vi "xml generate for SFP+_VNA_Full.vi"(0 "xmlPath":path=path "D:/wmgxml.xml", 5 "txtPath":path, 7 "singleItemInfo":T3[](array[typedef]), 9 "xml_detail":T2, 11 "TDD":T1) -> ()   [LabVIEW 2011]
uses:
  dataType/sSpec.ctl
  dataType/xml_detail.ctl
  dataType/TDD.ctl
  <vilib>/Utility/file.llb/Read From Spreadsheet File (DBL).vi
panel:
  out "FilePath":string
  out "FileVer":string
  out "Limit_NEXT":dbl[](array[numeric])
  out "Limit_SCC11":dbl[](array[numeric])
  out "Limit_SCD21-SDD21":dbl[](array[numeric])
  out "Limit_ILD":dbl[](array[numeric])
  out "Limit_SDD11":dbl[](array[numeric])
  out "limit_SDD21":dbl[](array[numeric])
  out "show_impspec":string[](array[string])
  out "terminal points 2":dbl[](array[numeric])
  in  "width2":dbl
  in  "width1":dbl
  out "TestResult":string
  out "cable points":dbl[](array[numeric])
  out "terminal points":dbl[](array[numeric])
  out "TDD":string
  out "NEXT":string
  out "SCC11":string
  out "SCD21-SDD21":string
  out "ILD":string
  out "SDD11":string
  out "SDD21":string
  out "midVar_time":string[](array[string])
  out "input_array_time":string[](array[string])
  out "input_str_CustomerPN":string
  in  "midVar_state":string
  in  "input_str_product":string
  out "input_str_label":string
  out "midVar_Content":string
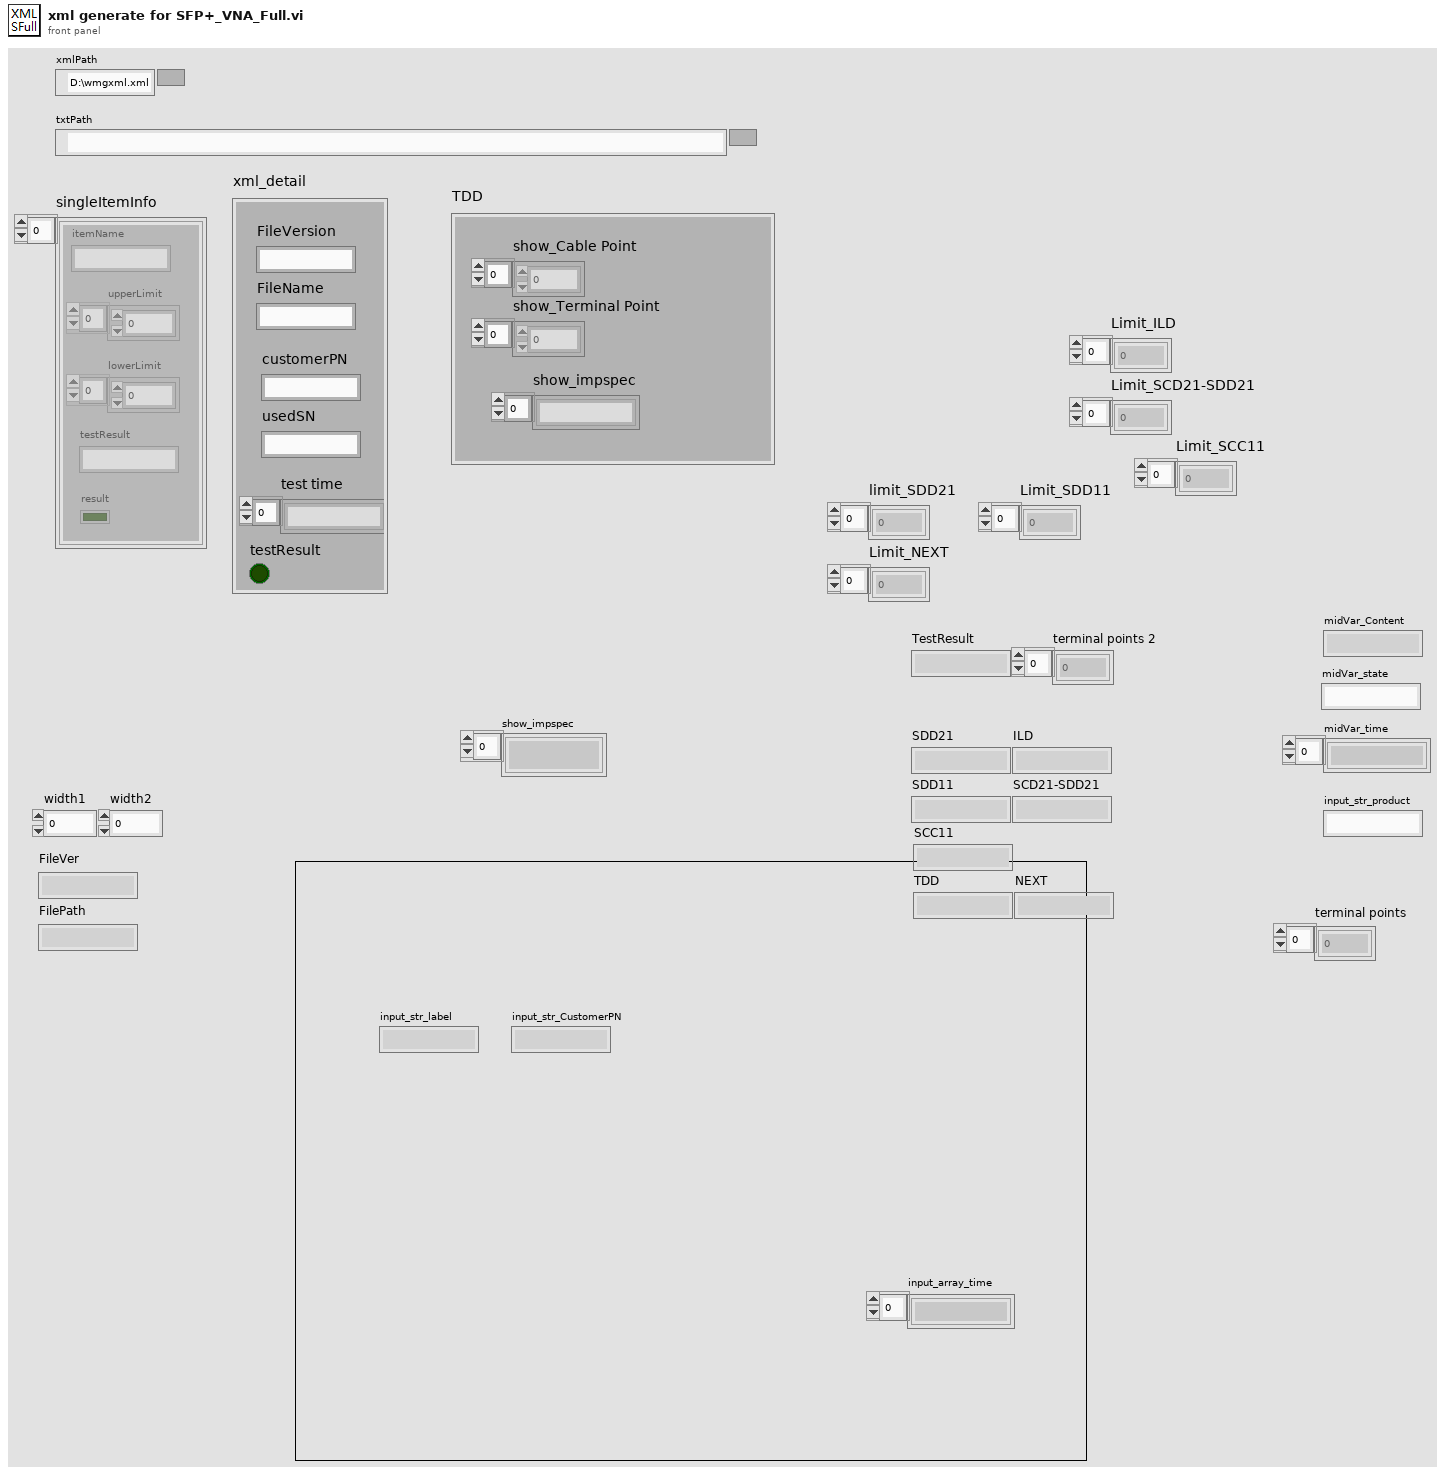
[diagram p1: front panel]
types:
  T1 = typedef "TDD.ctl" = cluster{"show_Cable Point":dbl[], "show_Terminal Point":dbl[], "show_impspec":string[]}
  T2 = typedef "xml_detail.ctl" = cluster{"FileVersion":string, "FileName":string, "customerPN":string, "usedSN":string, "test time":string[], "testResult":bool}
  T3 = typedef "sSpec.ctl" = cluster{"itemName":string, "upperLimit":dbl[], "lowerLimit":dbl[], "testResult":string, "result":bool}
  T4 = enum16{"open", "replace", "create", "open or create", "replace or create", "replace or create with confirmation"}
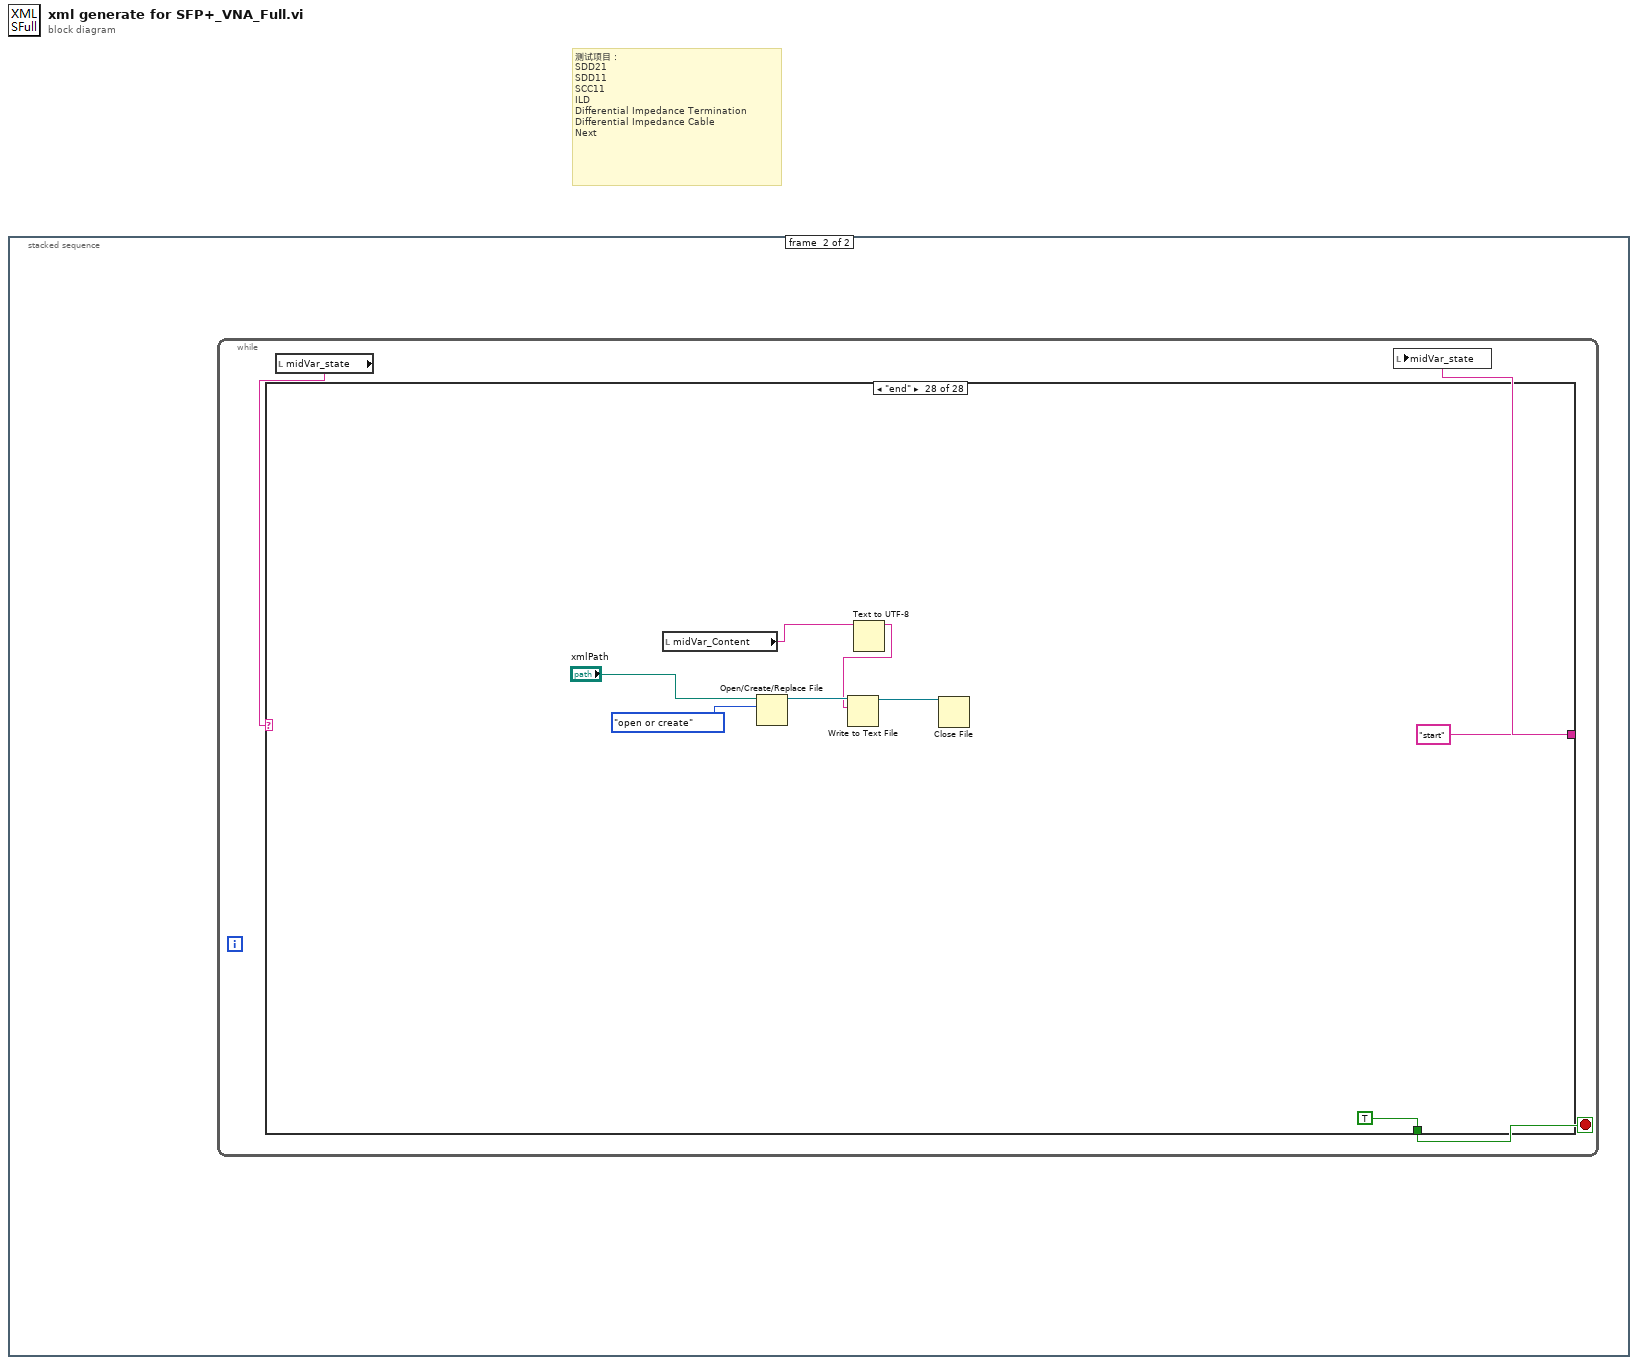
[diagram p0: block diagram]
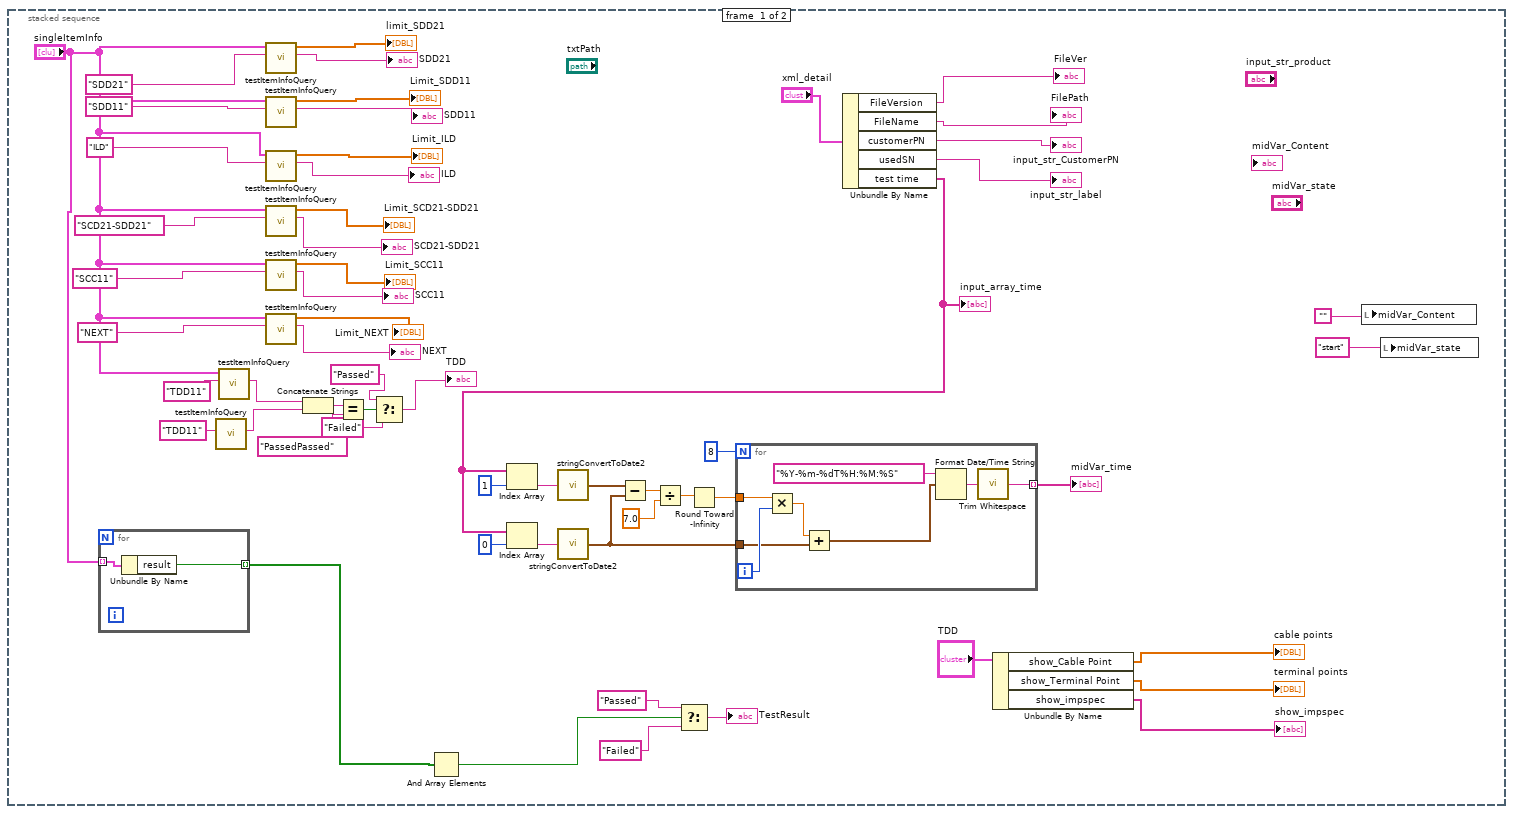
[diagram p2: hidden frame]
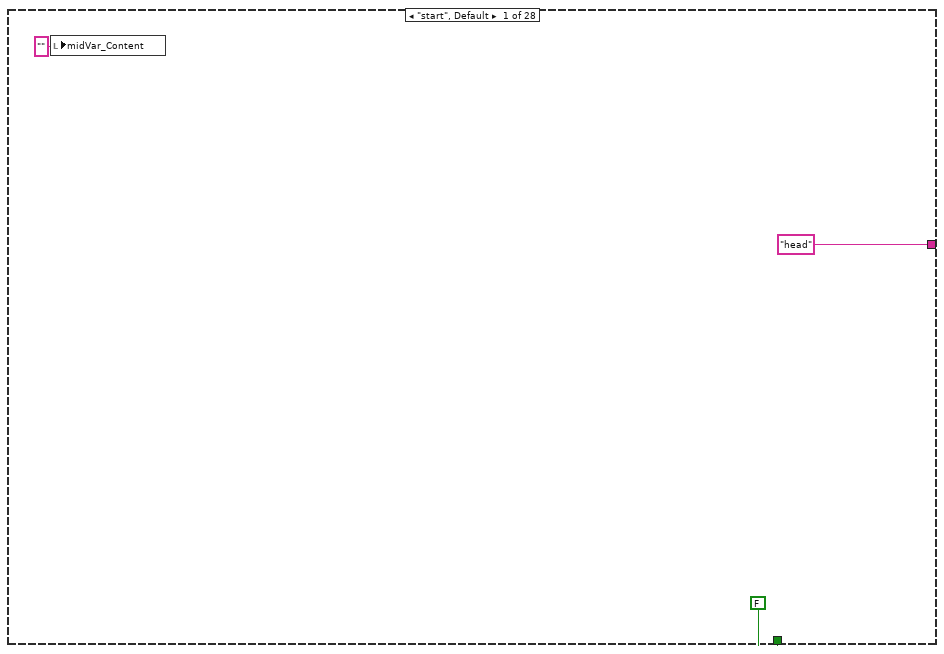
[diagram p3: hidden frame]
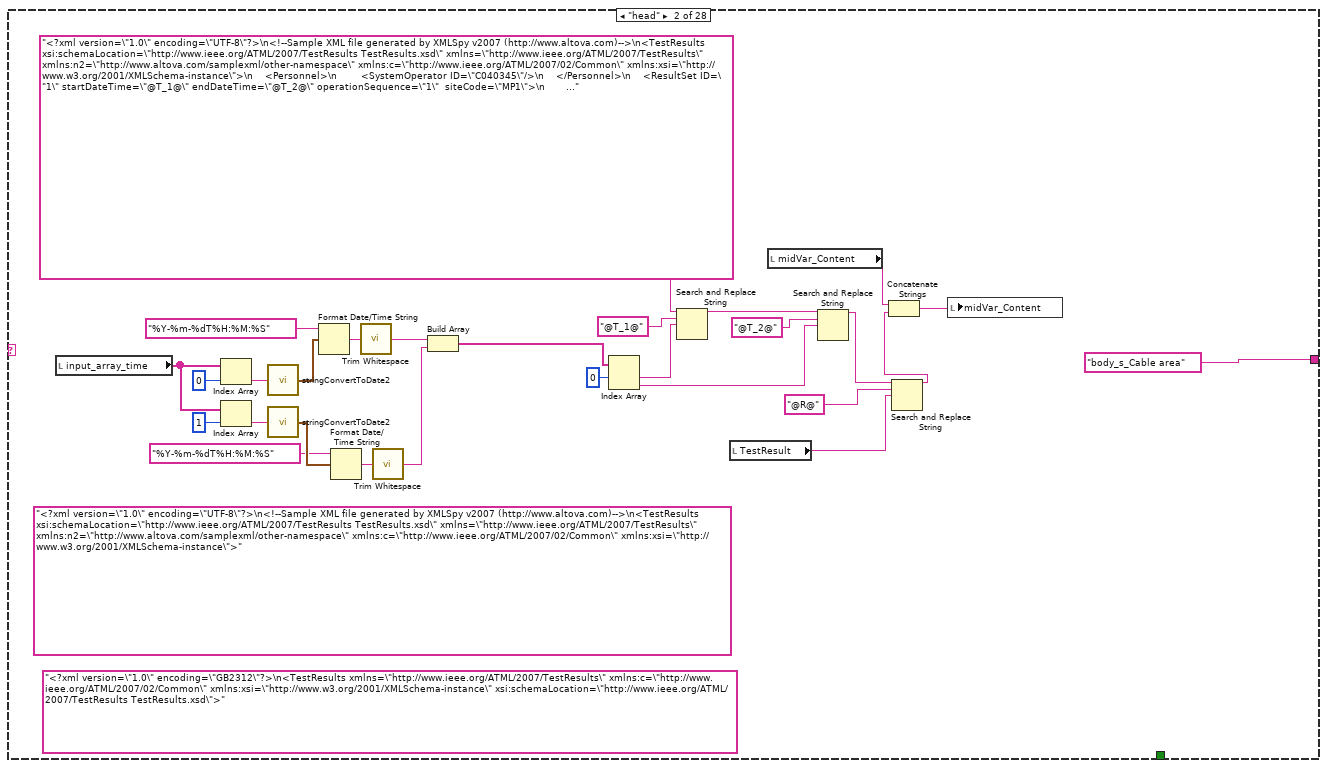
[diagram p4: hidden frame]
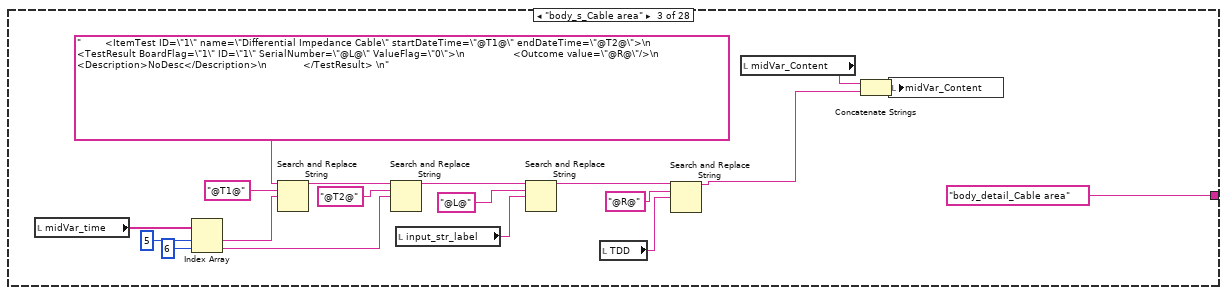
[diagram p5: hidden frame]
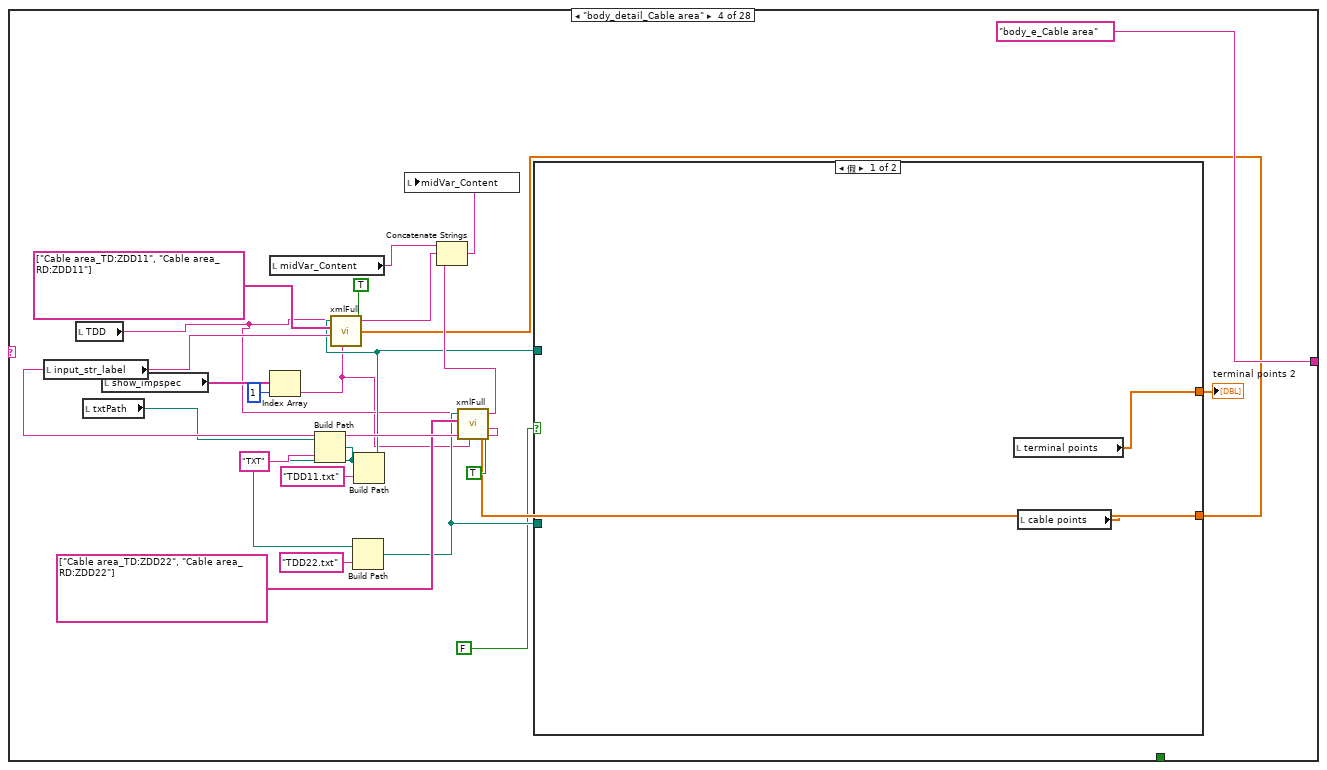
[diagram p6: hidden frame]
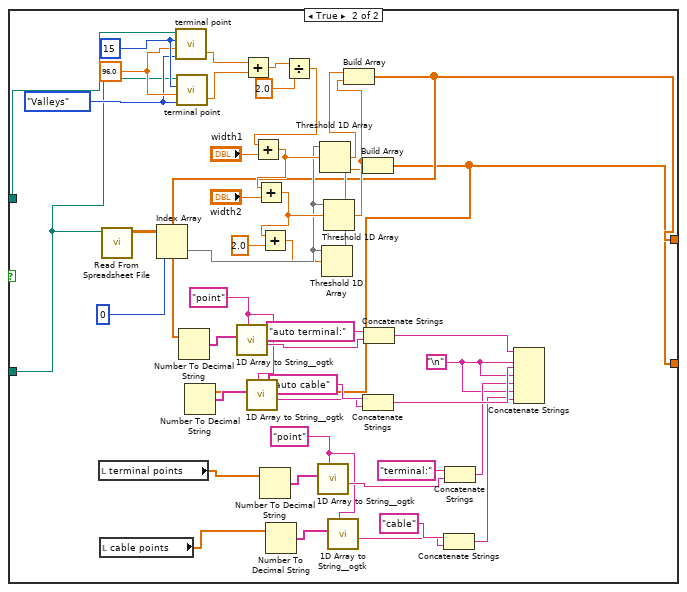
[diagram p7: hidden frame]
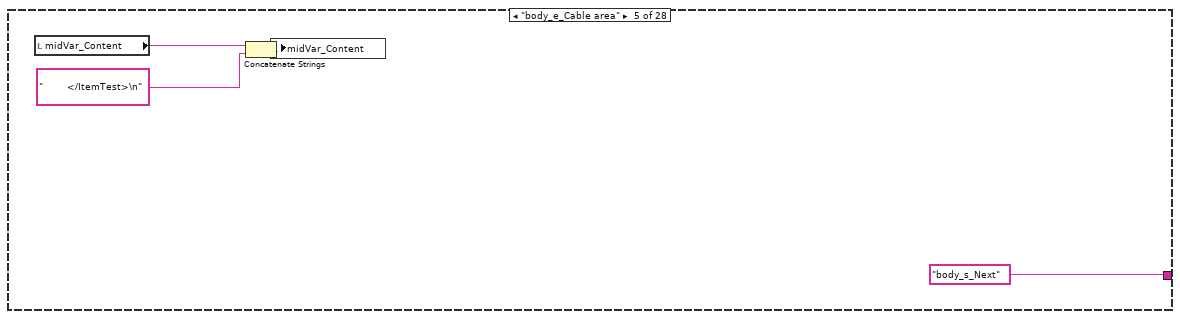
[diagram p8: hidden frame]
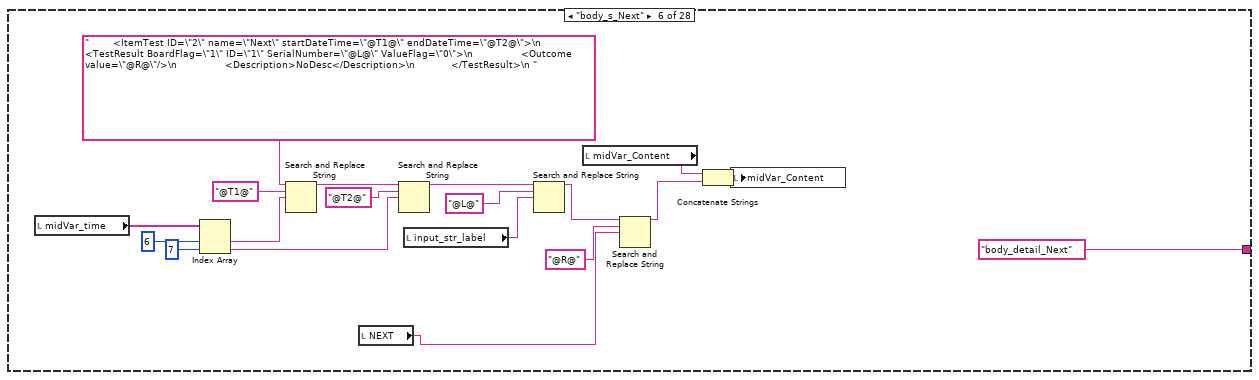
[diagram p9: hidden frame]
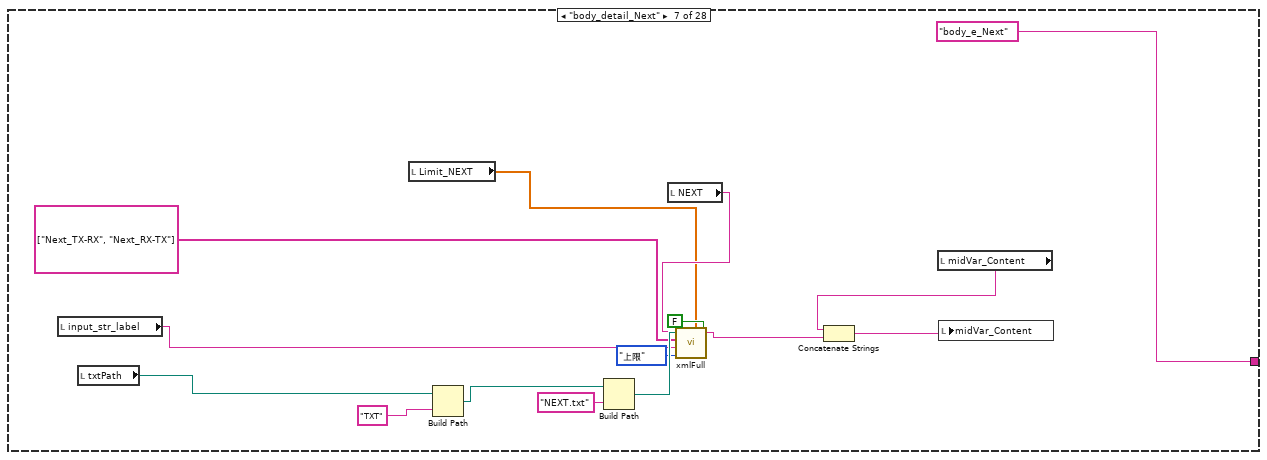
[diagram p10: hidden frame]
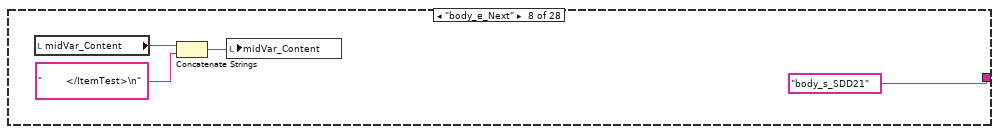
[diagram p11: hidden frame]
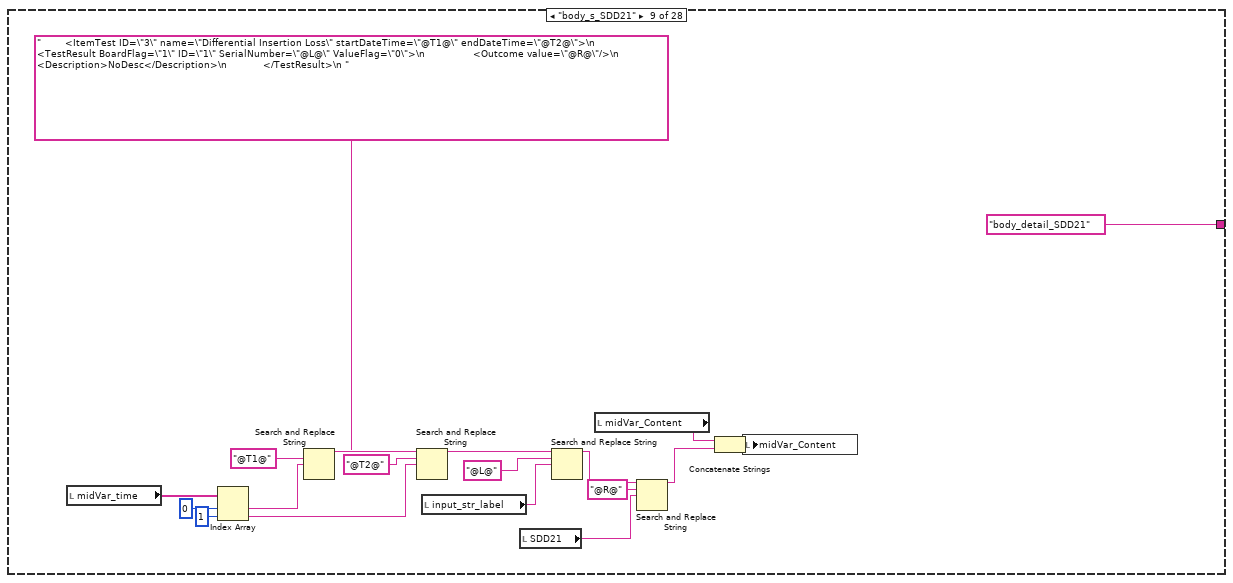
[diagram p12: hidden frame]
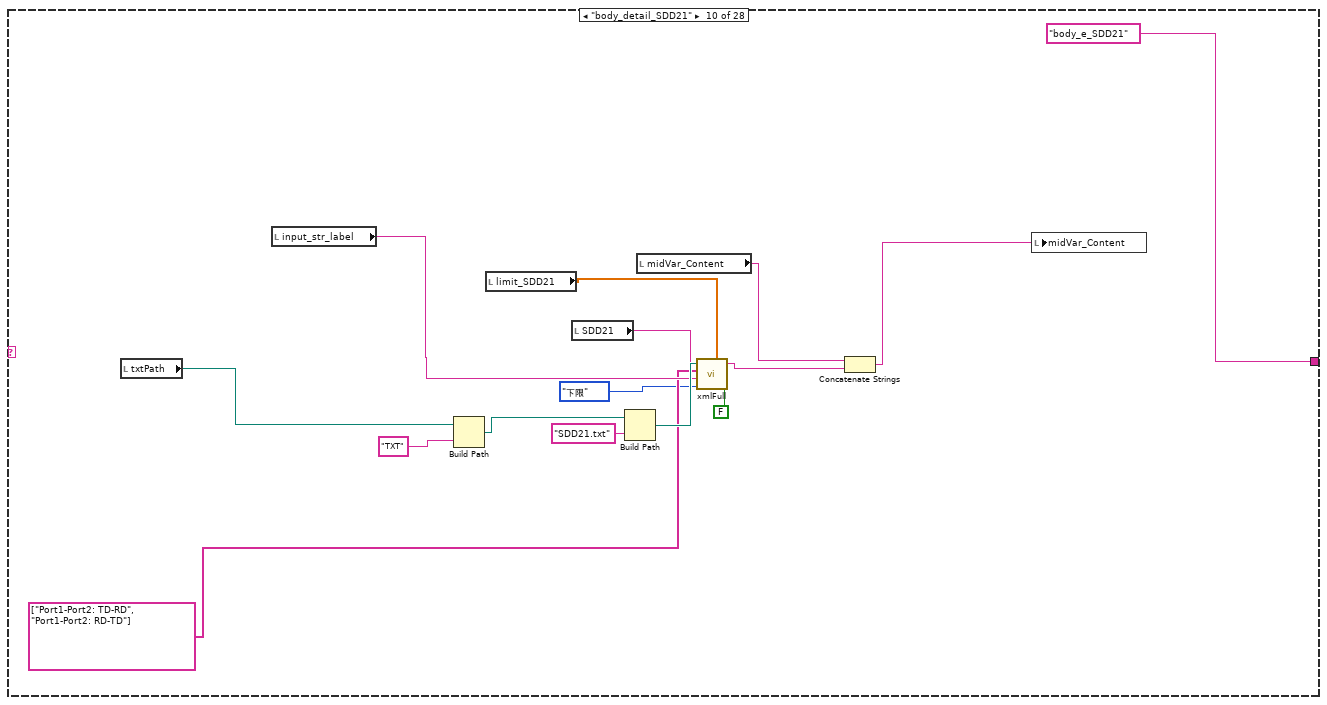
[diagram p13: hidden frame]
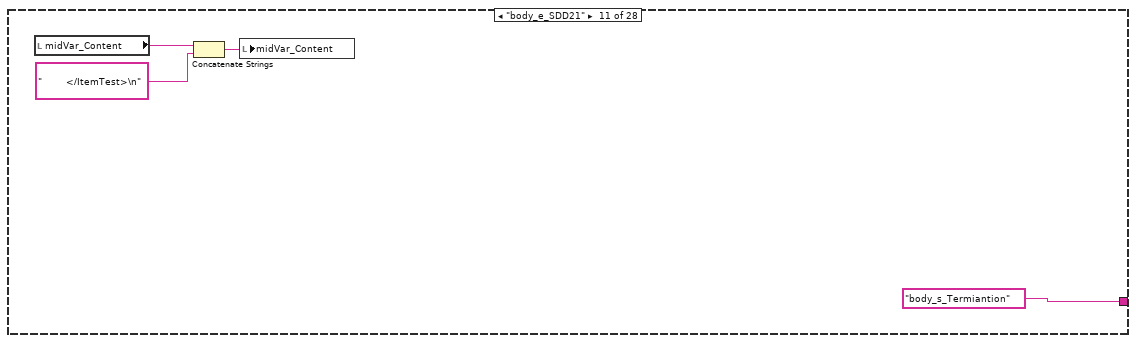
[diagram p14: hidden frame]
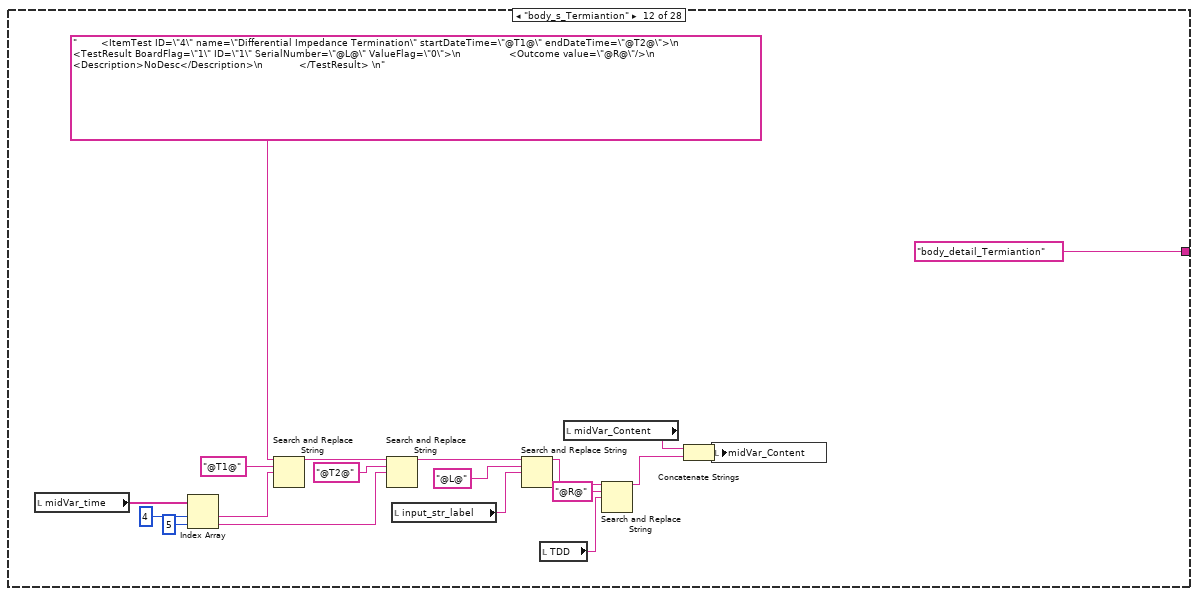
[diagram p15: hidden frame]
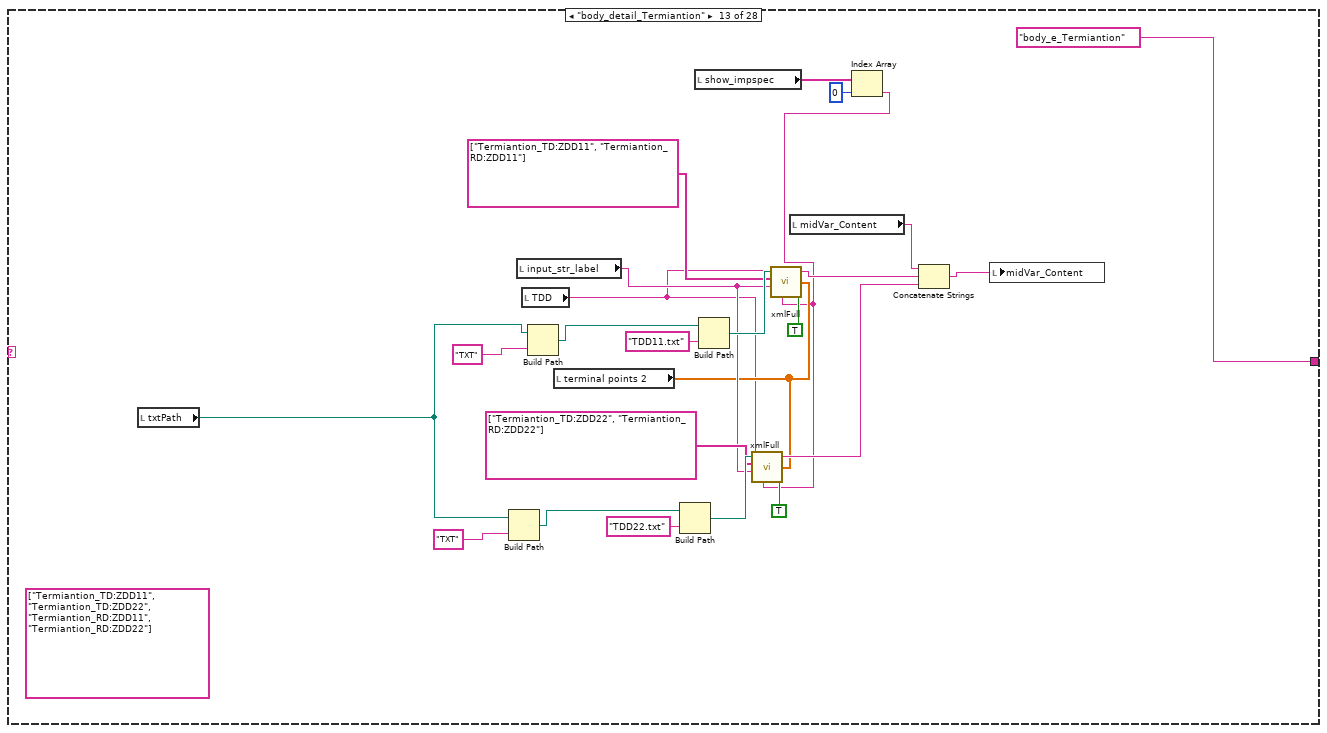
[diagram p16: hidden frame]
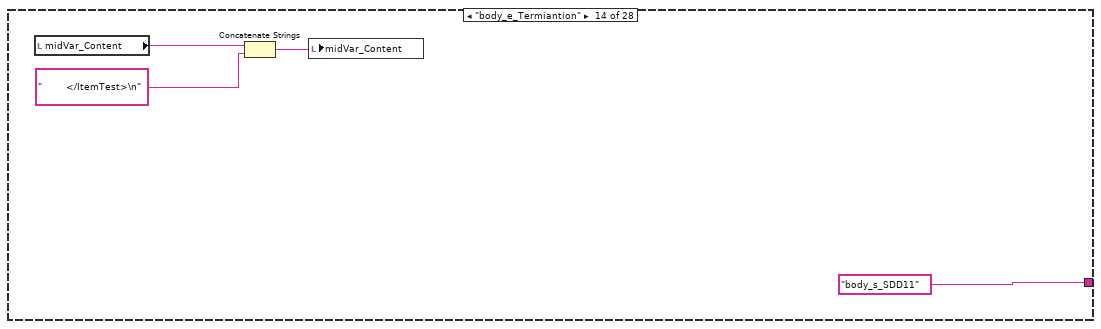
[diagram p17: hidden frame]
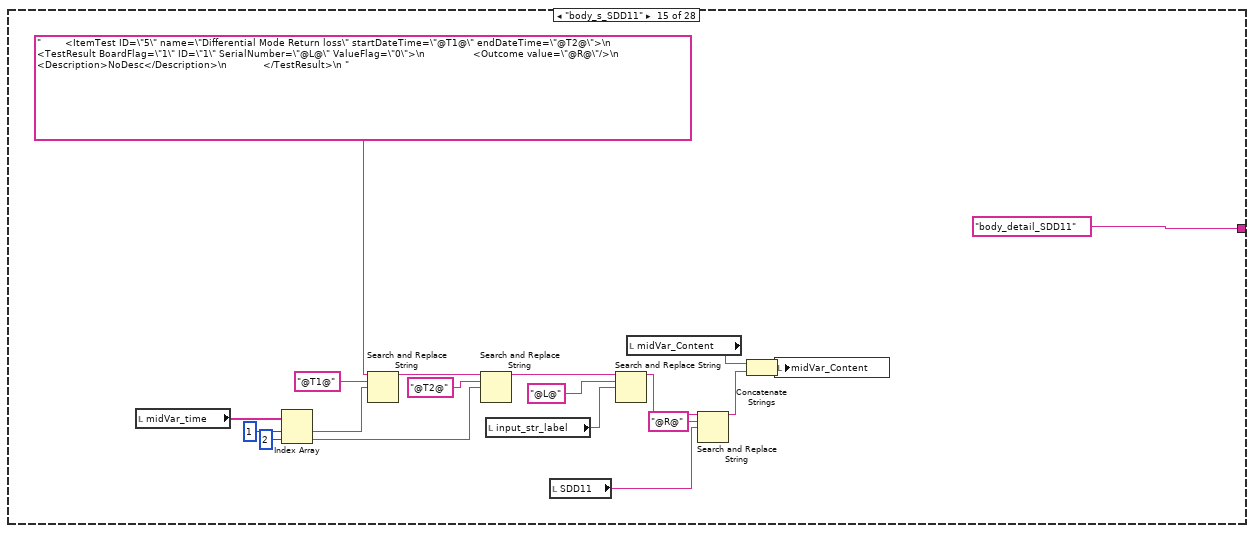
[diagram p18: hidden frame]
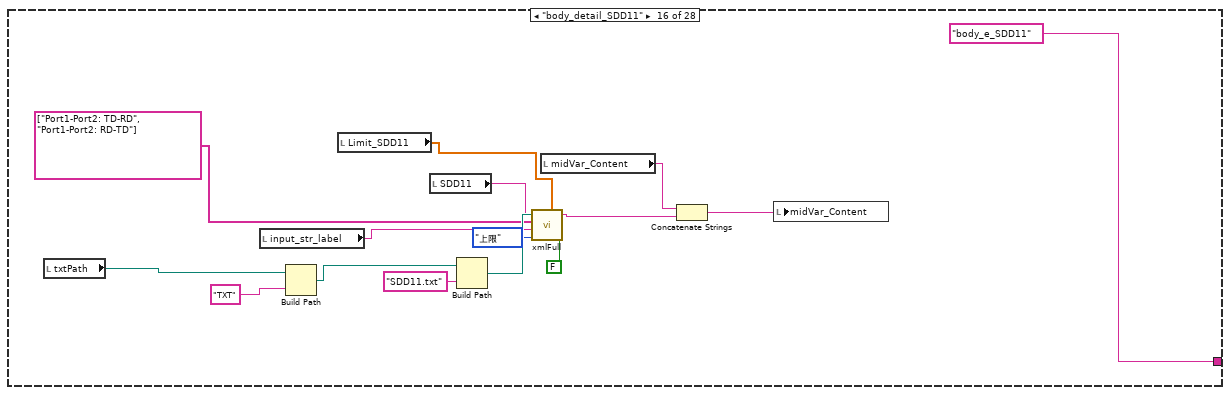
[diagram p19: hidden frame]
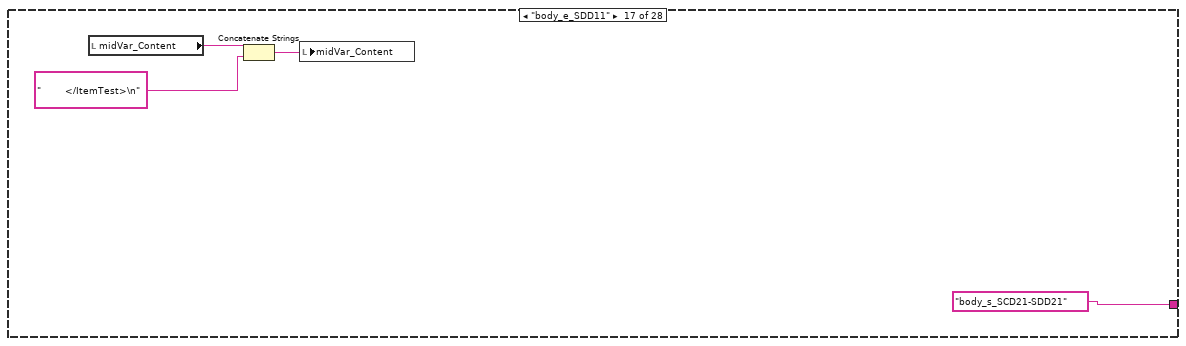
[diagram p20: hidden frame]
diagram:
  # "测试项目：\nSDD21\nSDD11\nSCC11\nILD\nDifferential Impedance Termination\nDifferential Impedance Cable\nNext"
  n1 = stacked-sequence {
    frame #0 {
      n2 = for {
        tunnel: "singleItemInfo" -> [w60] mode=indexing
        tunnel: [w59] -> w11 mode=indexing
        n3 = Unbundle By Name(w60) -> ("result"=w59:bool)
      }
      n4 = call "testItemInfoQuery.vi"("testItem"="TDD11") -> ("testResult"=w19:string)  [unwired: 9 in, 1 out]
      n5 = call "testItemInfoQuery.vi"("testItem"="TDD11", "singleItemInfo"="singleItemInfo") -> ("testResult"=w20:string)  [unwired: 8 in, 1 out]
      n6 = call "testItemInfoQuery.vi"("testItem"="SDD21", "singleItemInfo"="singleItemInfo") -> ("testResult"=→"SDD21":string, "Limit"=→"limit_SDD21":dbl[])  [unwired: 8 in]
      n7 = call "testItemInfoQuery.vi"("testItem"="SDD11", "singleItemInfo"="singleItemInfo") -> ("testResult"=→"SDD11":string, "Limit"=→"Limit_SDD11":dbl[])  [unwired: 8 in]
      n8 = call "testItemInfoQuery.vi"("testItem"="ILD", "singleItemInfo"="singleItemInfo") -> ("testResult"=→"ILD":string, "Limit"=→"Limit_ILD":dbl[])  [unwired: 8 in]
      n9 = call "testItemInfoQuery.vi"("testItem"="SCD21-SDD21", "singleItemInfo"="singleItemInfo") -> ("testResult"=→"SCD21-SDD21":string, "Limit"=→"Limit_SCD21-SDD21":dbl[])  [unwired: 8 in]
      n10 = call "testItemInfoQuery.vi"("testItem"="SCC11", "singleItemInfo"="singleItemInfo") -> ("testResult"=→"SCC11":string, "Limit"=→"Limit_SCC11":dbl[])  [unwired: 8 in]
      n11 = call "testItemInfoQuery.vi"("testItem"="NEXT", "singleItemInfo"="singleItemInfo") -> ("testResult"=→"NEXT":string, "Limit"=→"Limit_NEXT":dbl[])  [unwired: 8 in]
      n12 = Concatenate Strings(w20, w19) -> (w18:string)
      n13 = Equal?(x=w18, y="PassedPassed") -> (x = y?=w16:bool)
      n14 = Select(t="Passed", s=w16, f="Failed") -> (s? t:f=→"TDD":string)
      n15 = And Array Elements(Boolean array=w11) -> (logical AND=w42:bool)
      n16 = Select(t="Passed", s=w42, f="Failed") -> (s? t:f=→"TestResult":string)
      n17 = Unbundle By Name("xml_detail") -> ("FileVersion"=→"FileVer":string, "FileName"=→"FilePath":string, "customerPN"=→"input_str_CustomerPN":string, "usedSN"=→"input_str_label":string, "test time"=w5:string[])
      "input_array_time" <- w5
      n18 = Index Array(array=w5, index=1 ("索引")) -> (element=w47:string)
      n19 = Index Array(array=w5, index=0 ("索引")) -> (element=w48:string)
      n20 = call "stringConvertToDate2.vi"("input_str_yymmdd"=w47) -> ("show_date"=w49:timestamp)
      n21 = call "stringConvertToDate2.vi"("input_str_yymmdd"=w48) -> ("show_date"=w55:timestamp)
      n22 = Subtract(x=w49, y=w55) -> (x-y=w50:dbl)
      n23 = Divide(x=w50, y=7.0) -> (x/y=w52:dbl)
      n24 = Round Toward -Infinity(1:w52) -> (0:w54:dbl)
      n25 = for {
        N: 8 -> [_]
        tunnel: w54 -> [w68]
        tunnel: w55 -> [w66]
        tunnel: [w61] -> w56 mode=indexing
        i -> [w67]
        n26 = Multiply(x=w68, y=w67) -> (x*y=w65:dbl)
        n27 = Add(x=w65, y=w66) -> (x+y=w62:timestamp)
        n28 = Format Date/Time String(time format string (%c)="%Y-%m-%dT%H:%M:%S" ("时间格式字符串(%c)"), seconds (now)=w62) -> (date/time string=w63:string)  [unwired: 1 in]
        n29 = call <vilib>:"Trim Whitespace.vi"("string"=w63) -> ("trimmed string"=w61:string)  [unwired: 1 in]
      }
      "midVar_time" <- w56
      n30 = Unbundle By Name("TDD") -> ("show_Cable Point"=→"cable points":dbl[], "show_Terminal Point"=→"terminal points":dbl[], "show_impspec"=→"show_impspec":string[])
      n31 = local write "midVar_Content"("") -> ()
      n32 = local write "midVar_state"("start" ("state")) -> ()
    }
    frame #1 {
      n33 = while {
        stop <- w69 stop-if-true
        n34 = local read "midVar_state"() -> (w71:string)
        n35 = case shown="\"end\"" w71 {
          tunnel: ["head" ("state") "body_s_Cable area" ("state") "body_detail_Cable area" "body_e_Cable area" "body_s_Next" "body_detail_Next" "body_e_Next" "body_s_SDD21" "body_detail_SDD21" "body_e_SDD21" "body_s_Termiantion" "body_detail_Termiantion" "body_e_Termiantion" "body_s_SDD11" "body_detail_SDD11" "body_e_SDD11" "body_s_SCD21-SDD21" "body_detail_SCD21-SDD21" "body_e_SCD21-SDD21" "body_s_paddle card" "body_detail_paddle card" ("state") "body_e_paddle card" ("state") "body_s_ILD" ("state") "body_detail_ILD" "body_e_ILD" "tail" "end" ("state") "start" ("state")] -> w70
          tunnel: [FALSE _ _ _ _ _ _ _ _ _ _ _ _ _ _ _ _ _ _ _ _ _ _ _ _ _ _ TRUE] -> w69
          frame "start", Default {
            n36 = local write "midVar_Content"("" ("字符串")) -> ()
          }
          frame "head" {
            (unwired) "<?xml version=\"1.0\" encoding=\"GB2312\"?>\n<TestResults xmlns=\"http://www.ieee.org/ATML/2007/TestResults\" xmlns:c=\"http://www.ieee.org/ATML/2007/02/Common\" xmlns:xsi=\"http://www.w3.org/2001/XMLSchema-instance\" xsi:schemaLocation=\"http://www.ieee.org/ATML/2007/TestResults TestResults.xsd\">"
            (unwired) "<?xml version=\"1.0\" encoding=\"UTF-8\"?>\n<!--Sample XML file generated by XMLSpy v2007 (http://www.altova.com)-->\n<TestResults xsi:schemaLocation=\"http://www.ieee.org/ATML/2007/TestResults TestResults.xsd\" xmlns=\"http://www.ieee.org/ATML/2007/TestResults\" xmlns:n2=\"http://www.altova.com/samplexml/other-namespace\" xmlns:c=\"http://www.ieee.org/ATML/2007/02/Common\" xmlns:xsi=\"http://www.w3.org/2001/XMLSchema-instance\">"
            n37 = local read "input_array_time"() -> (w88:string[])
            n38 = Index Array(array=w88, index=0 ("索引")) -> (element=w87:string)
            n39 = Index Array(array=w88, index=1 ("索引")) -> (element=w86:string)
            n40 = call "stringConvertToDate2.vi"("input_str_yymmdd"=w87) -> ("show_date"=w84:timestamp)
            n41 = call "stringConvertToDate2.vi"("input_str_yymmdd"=w86) -> ("show_date"=w83:timestamp)
            n42 = Format Date/Time String(time format string (%c)="%Y-%m-%dT%H:%M:%S" ("时间格式字符串(%c)"), seconds (now)=w84) -> (date/time string=w91:string)  [unwired: 1 in]
            n43 = Format Date/Time String(time format string (%c)="%Y-%m-%dT%H:%M:%S" ("时间格式字符串(%c)"), seconds (now)=w83) -> (date/time string=w85:string)  [unwired: 1 in]
            n44 = call <vilib>:"Trim Whitespace.vi"("string"=w91) -> ("trimmed string"=w81:string)  [unwired: 1 in]
            n45 = call <vilib>:"Trim Whitespace.vi"("string"=w85) -> ("trimmed string"=w80:string)  [unwired: 1 in]
            n46 = Build Array(w81, w80) -> (w79:string[])
            n47 = Index Array(array=w79, index #1=0 ("索引")) -> (element #1=w100:string, element #2=w97:string)  [unwired: 1 in]
            n48 = Search and Replace String(input string="<?xml version=\"1.0\" encoding=\"UTF-8\"?>\n<!--Sample XML file generated by XMLSpy v2007 (http://www.altova.com)-->\n<TestResults xsi:schemaLocation=\"http://www.ieee.org/ATML/2007/TestResults TestResults.xsd\" xmlns=\"http://www.ieee.org/ATML/2007/TestResults\" xmlns:n2=\"http://www.altova.com/samplexml/other-namespace\" xmlns:c=\"http://www.ieee.org/ATML/2007/02/Common\" xmlns:xsi=\"http://www.w3.org/2001/XMLSchema-instance\">\n    <Personnel>\n        <SystemOperator ID=\"C040345\"/>\n    </Personnel>\n    <ResultSet ID=\"1\" startDateTime=\"@T_1@\" endDateTime=\"@T_2@\" operationSequence=\"1\"  siteCode=\"MP1\">\n        <Description>CMZ00A2R</Description>\n        <TestResult BoardFlag=\"1\" ID=\"1\">\n            <Outcome value=\"@R@\"/>\n        </TestResult>\n", search string="@T_1@" ("搜索字符串"), replace string=w100) -> (result string=w99:string)  [unwired: 5 in, 3 out]
            n49 = local read "TestResult"() -> (w75:string)
            n50 = local read "midVar_Content"() -> (w95:string)
            n51 = Search and Replace String(input string=w99, search string="@T_2@" ("搜索字符串"), replace string=w97) -> (result string=w78:string)  [unwired: 5 in, 3 out]
            n52 = Search and Replace String(input string=w78, search string="@R@" ("搜索字符串"), replace string=w75) -> (result string=w77:string)  [unwired: 5 in, 3 out]
            n53 = Concatenate Strings(w95, w77) -> (w94:string)
            n54 = local write "midVar_Content"(w94) -> ()
          }
          frame "body_s_Cable area" {
            n55 = local read "midVar_time"() -> (w108:string[])
            n56 = Index Array(array=w108, index #1=5 ("索引"), index #2=6 ("索引")) -> (element #1=w119:string, element #2=w116:string)
            n57 = Search and Replace String(input string="        <ItemTest ID=\"1\" name=\"Differential Impedance Cable\" startDateTime=\"@T1@\" endDateTime=\"@T2@\">\n            <TestResult BoardFlag=\"1\" ID=\"1\" SerialNumber=\"@L@\" ValueFlag=\"0\">\n                <Outcome value=\"@R@\"/>\n                <Description>NoDesc</Description>\n            </TestResult> \n", search string="@T1@" ("搜索字符串"), replace string=w119) -> (result string=w118:string)  [unwired: 5 in, 3 out]
            n58 = Search and Replace String(input string=w118, search string="@T2@" ("搜索字符串"), replace string=w116) -> (result string=w111:string)  [unwired: 5 in, 3 out]
            n59 = local read "input_str_label"() -> (w110:string)
            n60 = Search and Replace String(input string=w111, search string="@L@" ("搜索字符串"), replace string=w110) -> (result string=w106:string)  [unwired: 5 in, 3 out]
            n61 = local read "TDD"() -> (w103:string)
            n62 = Search and Replace String(input string=w106, search string="@R@" ("搜索字符串"), replace string=w103) -> (result string=w105:string)  [unwired: 5 in, 3 out]
            n63 = local read "midVar_Content"() -> (w115:string)
            n64 = Concatenate Strings(w115, w105) -> (w114:string)
            n65 = local write "midVar_Content"(w114) -> ()
          }
          frame "body_detail_Cable area" {
            n66 = local read "input_str_label"() -> (w137:string)
            n67 = local read "TDD"() -> (w124:string)
            n68 = local read "txtPath"() -> (w134:path)
            n69 = local read "show_impspec"() -> (w126:string[])
            n70 = local read "midVar_Content"() -> (w144:string)
            n71 = Index Array(array=w126, index=1 ("索引")) -> (element=w123:string)
            n72 = Build Path(base path=w134, name or relative path="TXT" ("名称或相对路径")) -> (appended path=w133:path)
            n73 = Build Path(base path=w133, name or relative path="TDD22.txt" ("名称或相对路径")) -> (appended path=w130:path)
            n74 = Build Path(base path=w133, name or relative path="TDD11.txt" ("名称或相对路径")) -> (appended path=w129:path)
            n75 = case shown="假" FALSE ("auto get refer point") {
              tunnel: w130 -> [_ w180]
              tunnel: w129 -> [_ w192]
              tunnel: [w146 w153] -> w127
              tunnel: [w147 w154] -> w128
              frame False {
                n76 = local read "terminal points"() -> (w147:dbl[])
                n77 = local read "cable points"() -> (w146:dbl[])
              }
              frame True {
                w149 = "\n"
                w157 = "point" ("delimiter (Tab)")
                w166 = "point" ("delimiter (Tab)")
                w189 = enum32{"Peaks", "Valleys"}."Valleys" ("peaks/valleys")
                w190 = 96.0 ("threshold")
                w191 = 15 ("PD width")
                n78 = local read "terminal points"() -> (w162:dbl[])
                n79 = local read "cable points"() -> (w163:dbl[])
                n80 = call-poly <vilib>:"Read From Spreadsheet File.vi"("file path (dialog if empty)"=w180) -> ("all rows"=w179:dbl[][])  [unwired: 6 in, 4 out]
                n81 = Index Array(array=w179, index (col)=0 ("禁用的索引 (列)")) -> (element=w175:dbl[])  [unwired: 1 in]
                n82 = call "terminal point.vi"("peaks/valleys"=w189, "threshold"=w190, "PD width"=w191, "TDD filePath"=w192) -> ("time low"=w184:dbl)  [unwired: 1 out]
                n83 = call "terminal point.vi"("peaks/valleys"=w189, "threshold"=w190, "PD width"=w191, "TDD filePath"=w180) -> ("time low"=w183:dbl)  [unwired: 1 out]
                n84 = Add(x=w184, y=w183) -> (x+y=w188:dbl)
                n85 = Number To Decimal String(number=w162) -> (decimal integer string=w164:string[])  [unwired: 1 in]
                n86 = Number To Decimal String(number=w163) -> (decimal integer string=w165:string[])  [unwired: 1 in]
                n87 = Divide(x=w188, y=2.0) -> (x/y=w181:dbl)
                n88 = Add(x=w181, y="width1") -> (x+y=w177:dbl)
                n89 = Add(x=w177, y="width2") -> (x+y=w176:dbl)
                n90 = Add(x=w176, y=2.0) -> (x+y=w174:dbl)
                n91 = call <userlib>:"1D Array to String__ogtk.vi"("delimiter (Tab)"=w166, "Array of Strings"=w164) -> ("delimited string"=w168:string)  [unwired: 9 in]
                n92 = Threshold 1D Array(2:w177, 3:w175) -> (0:w173:dbl)  [unwired: 1 in]
                n93 = Threshold 1D Array(2:w174, 3:w175) -> (0:w171:dbl)  [unwired: 1 in]
                n94 = Threshold 1D Array(2:w176, 3:w175) -> (0:w172:dbl)  [unwired: 1 in]
                n95 = call <userlib>:"1D Array to String__ogtk.vi"("delimiter (Tab)"=w166, "Array of Strings"=w165) -> ("delimited string"=w169:string)  [unwired: 9 in]
                n96 = Build Array(w173, w172) -> (w154:dbl[])
                n97 = Number To Decimal String(number=w154) -> (decimal integer string=w155:string[])  [unwired: 1 in]
                n98 = call <userlib>:"1D Array to String__ogtk.vi"("delimiter (Tab)"=w157, "Array of Strings"=w155) -> ("delimited string"=w159:string)  [unwired: 9 in]
                n99 = Build Array(w172, w171) -> (w153:dbl[])
                n100 = Number To Decimal String(number=w153) -> (decimal integer string=w156:string[])  [unwired: 1 in]
                n101 = call <userlib>:"1D Array to String__ogtk.vi"("delimiter (Tab)"=w157, "Array of Strings"=w156) -> ("delimited string"=w160:string)  [unwired: 9 in]
                n102 = Concatenate Strings("auto cable" ("字符串"), w160) -> (w151:string)
                n103 = Concatenate Strings("auto terminal:" ("字符串"), w159) -> (w152:string)
                n104 = Concatenate Strings("cable" ("字符串"), w169) -> (w148:string)
                n105 = Concatenate Strings("terminal:" ("字符串"), w168) -> (w150:string)
                n106 = Concatenate Strings(w152, w149, w151, w149, w150, w149, w148) -> ()  [unwired: 1 out]
              }
            }
            "terminal points 2" <- w128
            n107 = call "xmlFull.vi"("TDD?"=TRUE, "Points"=w127, "file path (dialog if empty)"=w129, "TDD spec"=w123, "SN"=w137, "数组"=string[] ["Cable area_TD:ZDD11", "Cable area_RD:ZDD11"], "second result"=w124) -> ("OutPutXml"=w142:string)  [unwired: 3 in]
            n108 = call "xmlFull.vi"("TDD?"=TRUE, "Points"=w127, "file path (dialog if empty)"=w130, "TDD spec"=w123, "SN"=w137, "数组"=string[] ["Cable area_TD:ZDD22", "Cable area_RD:ZDD22"], "second result"=w124) -> ("OutPutXml"=w135:string)  [unwired: 3 in]
            n109 = Concatenate Strings(w144, w142, w135) -> (w143:string)
            n110 = local write "midVar_Content"(w143) -> ()
          }
          frame "body_e_Cable area" {
            n111 = local read "midVar_Content"() -> (w196:string)
            n112 = Concatenate Strings(w196, "        </ItemTest>\n") -> (w195:string)
            n113 = local write "midVar_Content"(w195) -> ()
          }
          frame "body_s_Next" {
            n114 = local read "midVar_time"() -> (w202:string[])
            n115 = Index Array(array=w202, index #1=6 ("索引"), index #2=7 ("索引")) -> (element #1=w213:string, element #2=w210:string)
            n116 = Search and Replace String(input string="        <ItemTest ID=\"2\" name=\"Next\" startDateTime=\"@T1@\" endDateTime=\"@T2@\">\n            <TestResult BoardFlag=\"1\" ID=\"1\" SerialNumber=\"@L@\" ValueFlag=\"0\">\n                <Outcome value=\"@R@\"/>\n                <Description>NoDesc</Description>\n            </TestResult>\n ", search string="@T1@" ("搜索字符串"), replace string=w213) -> (result string=w212:string)  [unwired: 5 in, 3 out]
            n117 = local read "NEXT"() -> (w200:string)
            n118 = Search and Replace String(input string=w212, search string="@T2@" ("搜索字符串"), replace string=w210) -> (result string=w205:string)  [unwired: 5 in, 3 out]
            n119 = local read "input_str_label"() -> (w204:string)
            n120 = Search and Replace String(input string=w205, search string="@L@" ("搜索字符串"), replace string=w204) -> (result string=w198:string)  [unwired: 5 in, 3 out]
            n121 = local read "midVar_Content"() -> (w209:string)
            n122 = Search and Replace String(input string=w198, search string="@R@" ("搜索字符串"), replace string=w200) -> (result string=w197:string)  [unwired: 5 in, 3 out]
            n123 = Concatenate Strings(w209, w197) -> (w208:string)
            n124 = local write "midVar_Content"(w208) -> ()
          }
          frame "body_detail_Next" {
            n125 = local read "input_str_label"() -> (w224:string)
            n126 = local read "txtPath"() -> (w226:path)
            n127 = local read "Limit_NEXT"() -> (w216:dbl[])
            n128 = Build Path(base path=w226, name or relative path="TXT" ("名称或相对路径")) -> (appended path=w228:path)
            n129 = Build Path(base path=w228, name or relative path="NEXT.txt" ("名称或相对路径")) -> (appended path=w225:path)
            n130 = local read "NEXT"() -> (w218:string)
            n131 = call "xmlFull.vi"("TDD?"=FALSE, "single spec"=w216, "file path (dialog if empty)"=w225, "limit type"=enum16{"上限", "下限"}."上限", "SN"=w224, "数组"=string[] ["Next_TX-RX", "Next_RX-TX"], "second result"=w218) -> ("OutPutXml"=w222:string)  [unwired: 3 in]
            n132 = local read "midVar_Content"() -> (w221:string)
            n133 = Concatenate Strings(w221, w222) -> (w220:string)
            n134 = local write "midVar_Content"(w220) -> ()
          }
          frame "body_e_Next" {
            n135 = local read "midVar_Content"() -> (w234:string)
            n136 = Concatenate Strings(w234, "        </ItemTest>\n") -> (w233:string)
            n137 = local write "midVar_Content"(w233) -> ()
          }
          frame "body_s_SDD21" {
            n138 = local read "midVar_time"() -> (w240:string[])
            n139 = Index Array(array=w240, index #1=0 ("索引"), index #2=1 ("索引")) -> (element #1=w251:string, element #2=w248:string)
            n140 = Search and Replace String(input string="        <ItemTest ID=\"3\" name=\"Differential Insertion Loss\" startDateTime=\"@T1@\" endDateTime=\"@T2@\">\n            <TestResult BoardFlag=\"1\" ID=\"1\" SerialNumber=\"@L@\" ValueFlag=\"0\">\n                <Outcome value=\"@R@\"/>\n                <Description>NoDesc</Description>\n            </TestResult>\n ", search string="@T1@" ("搜索字符串"), replace string=w251) -> (result string=w250:string)  [unwired: 5 in, 3 out]
            n141 = Search and Replace String(input string=w250, search string="@T2@" ("搜索字符串"), replace string=w248) -> (result string=w243:string)  [unwired: 5 in, 3 out]
            n142 = local read "input_str_label"() -> (w242:string)
            n143 = local read "SDD21"() -> (w235:string)
            n144 = Search and Replace String(input string=w243, search string="@L@" ("搜索字符串"), replace string=w242) -> (result string=w238:string)  [unwired: 5 in, 3 out]
            n145 = local read "midVar_Content"() -> (w247:string)
            n146 = Search and Replace String(input string=w238, search string="@R@" ("搜索字符串"), replace string=w235) -> (result string=w237:string)  [unwired: 5 in, 3 out]
            n147 = Concatenate Strings(w247, w237) -> (w246:string)
            n148 = local write "midVar_Content"(w246) -> ()
          }
          frame "body_detail_SDD21" {
            n149 = local read "txtPath"() -> (w262:path)
            n150 = local read "input_str_label"() -> (w261:string)
            n151 = Build Path(base path=w262, name or relative path="TXT" ("名称或相对路径")) -> (appended path=w266:path)
            n152 = local read "limit_SDD21"() -> (w254:dbl[])
            n153 = local read "SDD21"() -> (w256:string)
            n154 = Build Path(base path=w266, name or relative path="SDD21.txt" ("名称或相对路径")) -> (appended path=w264:path)
            n155 = local read "midVar_Content"() -> (w259:string)
            n156 = call "xmlFull.vi"("TDD?"=FALSE, "single spec"=w254, "file path (dialog if empty)"=w264, "limit type"=enum16{"上限", "下限"}."下限", "SN"=w261, "数组"=string[] ["Port1-Port2: TD-RD", "Port1-Port2: RD-TD"], "second result"=w256) -> ("OutPutXml"=w263:string)  [unwired: 3 in]
            n157 = Concatenate Strings(w259, w263) -> (w260:string)
            n158 = local write "midVar_Content"(w260) -> ()
          }
          frame "body_e_SDD21" {
            n159 = local read "midVar_Content"() -> (w272:string)
            n160 = Concatenate Strings(w272, "        </ItemTest>\n") -> (w271:string)
            n161 = local write "midVar_Content"(w271) -> ()
          }
          frame "body_s_Termiantion" {
            n162 = local read "midVar_time"() -> (w278:string[])
            n163 = Index Array(array=w278, index #1=4 ("索引"), index #2=5 ("索引")) -> (element #1=w289:string, element #2=w286:string)
            n164 = Search and Replace String(input string="        <ItemTest ID=\"4\" name=\"Differential Impedance Termination\" startDateTime=\"@T1@\" endDateTime=\"@T2@\">\n            <TestResult BoardFlag=\"1\" ID=\"1\" SerialNumber=\"@L@\" ValueFlag=\"0\">\n                <Outcome value=\"@R@\"/>\n                <Description>NoDesc</Description>\n            </TestResult> \n", search string="@T1@" ("搜索字符串"), replace string=w289) -> (result string=w288:string)  [unwired: 5 in, 3 out]
            n165 = Search and Replace String(input string=w288, search string="@T2@" ("搜索字符串"), replace string=w286) -> (result string=w281:string)  [unwired: 5 in, 3 out]
            n166 = local read "input_str_label"() -> (w280:string)
            n167 = Search and Replace String(input string=w281, search string="@L@" ("搜索字符串"), replace string=w280) -> (result string=w276:string)  [unwired: 5 in, 3 out]
            n168 = local read "TDD"() -> (w273:string)
            n169 = local read "midVar_Content"() -> (w285:string)
            n170 = Search and Replace String(input string=w276, search string="@R@" ("搜索字符串"), replace string=w273) -> (result string=w275:string)  [unwired: 5 in, 3 out]
            n171 = Concatenate Strings(w285, w275) -> (w284:string)
            n172 = local write "midVar_Content"(w284) -> ()
          }
          frame "body_detail_Termiantion" {
            (unwired) string[] ["Termiantion_TD:ZDD11", "Termiantion_TD:ZDD22", "Termiantion_RD:ZDD11", "Termiantion_RD:ZDD22"]
            n173 = local read "txtPath"() -> (w302:path)
            n174 = Build Path(base path=w302, name or relative path="TXT" ("名称或相对路径")) -> (appended path=w309:path)
            n175 = local read "input_str_label"() -> (w299:string)
            n176 = local read "TDD"() -> (w295:string)
            n177 = Build Path(base path=w302, name or relative path="TXT" ("名称或相对路径")) -> (appended path=w313:path)
            n178 = local read "terminal points 2"() -> (w296:dbl[])
            n179 = Build Path(base path=w309, name or relative path="TDD22.txt" ("名称或相对路径")) -> (appended path=w307:path)
            n180 = local read "show_impspec"() -> (w294:string[])
            n181 = Build Path(base path=w313, name or relative path="TDD11.txt" ("名称或相对路径")) -> (appended path=w311:path)
            n182 = local read "midVar_Content"() -> (w297:string)
            n183 = Index Array(array=w294, index=0 ("索引")) -> (element=w292:string)
            n184 = call "xmlFull.vi"("TDD?"=TRUE, "Points"=w296, "file path (dialog if empty)"=w307, "TDD spec"=w292, "SN"=w299, "数组"=string[] ["Termiantion_TD:ZDD22", "Termiantion_RD:ZDD22"], "second result"=w295) -> ("OutPutXml"=w305:string)  [unwired: 3 in]
            n185 = call "xmlFull.vi"("TDD?"=TRUE, "Points"=w296, "file path (dialog if empty)"=w311, "TDD spec"=w292, "SN"=w299, "数组"=string[] ["Termiantion_TD:ZDD11", "Termiantion_RD:ZDD11"], "second result"=w295) -> ("OutPutXml"=w306:string)  [unwired: 3 in]
            n186 = Concatenate Strings(w297, w306, w305) -> (w298:string)
            n187 = local write "midVar_Content"(w298) -> ()
          }
          frame "body_e_Termiantion" {
            n188 = local read "midVar_Content"() -> (w319:string)
            n189 = Concatenate Strings(w319, "        </ItemTest>\n") -> (w318:string)
            n190 = local write "midVar_Content"(w318) -> ()
          }
          frame "body_s_SDD11" {
            n191 = local read "midVar_time"() -> (w325:string[])
            n192 = Index Array(array=w325, index #1=1 ("索引"), index #2=2 ("索引")) -> (element #1=w336:string, element #2=w333:string)
            n193 = Search and Replace String(input string="        <ItemTest ID=\"5\" name=\"Differential Mode Return loss\" startDateTime=\"@T1@\" endDateTime=\"@T2@\">\n            <TestResult BoardFlag=\"1\" ID=\"1\" SerialNumber=\"@L@\" ValueFlag=\"0\">\n                <Outcome value=\"@R@\"/>\n                <Description>NoDesc</Description>\n            </TestResult>\n ", search string="@T1@" ("搜索字符串"), replace string=w336) -> (result string=w335:string)  [unwired: 5 in, 3 out]
            n194 = Search and Replace String(input string=w335, search string="@T2@" ("搜索字符串"), replace string=w333) -> (result string=w328:string)  [unwired: 5 in, 3 out]
            n195 = local read "input_str_label"() -> (w327:string)
            n196 = local read "SDD11"() -> (w320:string)
            n197 = Search and Replace String(input string=w328, search string="@L@" ("搜索字符串"), replace string=w327) -> (result string=w323:string)  [unwired: 5 in, 3 out]
            n198 = local read "midVar_Content"() -> (w332:string)
            n199 = Search and Replace String(input string=w323, search string="@R@" ("搜索字符串"), replace string=w320) -> (result string=w322:string)  [unwired: 5 in, 3 out]
            n200 = Concatenate Strings(w332, w322) -> (w331:string)
            n201 = local write "midVar_Content"(w331) -> ()
          }
          frame "body_detail_SDD11" {
            n202 = local read "txtPath"() -> (w342:path)
            n203 = local read "input_str_label"() -> (w345:string)
            n204 = Build Path(base path=w342, name or relative path="TXT" ("名称或相对路径")) -> (appended path=w351:path)
            n205 = local read "Limit_SDD11"() -> (w339:dbl[])
            n206 = local read "SDD11"() -> (w341:string)
            n207 = Build Path(base path=w351, name or relative path="SDD11.txt" ("名称或相对路径")) -> (appended path=w349:path)
            n208 = call "xmlFull.vi"("TDD?"=FALSE, "single spec"=w339, "file path (dialog if empty)"=w349, "limit type"=enum16{"上限", "下限"}."上限", "SN"=w345, "数组"=string[] ["Port1-Port2: TD-RD", "Port1-Port2: RD-TD"], "second result"=w341) -> ("OutPutXml"=w348:string)  [unwired: 3 in]
            n209 = local read "midVar_Content"() -> (w344:string)
            n210 = Concatenate Strings(w344, w348) -> (w343:string)
            n211 = local write "midVar_Content"(w343) -> ()
          }
          frame "body_e_SDD11" {
            n212 = local read "midVar_Content"() -> (w357:string)
            n213 = Concatenate Strings(w357, "        </ItemTest>\n") -> (w356:string)
            n214 = local write "midVar_Content"(w356) -> ()
          }
          frame "body_s_SCD21-SDD21" {
            n215 = local read "midVar_time"() -> (w363:string[])
            n216 = local read "input_str_label"() -> (w365:string)
            n217 = Index Array(array=w363, index #1=2 ("索引"), index #2=3 ("索引")) -> (element #1=w374:string, element #2=w371:string)
            n218 = Search and Replace String(input string="        <ItemTest ID=\"6\" name=\"Jitter From (SCD21-SDD21)\" startDateTime=\"@T1@\" endDateTime=\"@T2@\">\n            <TestResult BoardFlag=\"1\" ID=\"1\" SerialNumber=\"@L@\" ValueFlag=\"0\">\n                <Outcome value=\"@R@\"/>\n                <Description>NoDesc</Description>\n            </TestResult>\n ", search string="@T1@" ("搜索字符串"), replace string=w374) -> (result string=w373:string)  [unwired: 5 in, 3 out]
            n219 = Search and Replace String(input string=w373, search string="@T2@" ("搜索字符串"), replace string=w371) -> (result string=w366:string)  [unwired: 5 in, 3 out]
            n220 = Search and Replace String(input string=w366, search string="@L@" ("搜索字符串"), replace string=w365) -> (result string=w361:string)  [unwired: 5 in, 3 out]
            n221 = local read "SCD21-SDD21"() -> (w358:string)
            n222 = Search and Replace String(input string=w361, search string="@R@" ("搜索字符串"), replace string=w358) -> (result string=w360:string)  [unwired: 5 in, 3 out]
            n223 = local read "midVar_Content"() -> (w370:string)
            n224 = Concatenate Strings(w370, w360) -> (w369:string)
            n225 = local write "midVar_Content"(w369) -> ()
          }
          frame "body_detail_SCD21-SDD21" {
            n226 = local read "txtPath"() -> (w384:path)
            n227 = local read "SCD21-SDD21"() -> (w379:string)
            n228 = local read "input_str_label"() -> (w383:string)
            n229 = Build Path(base path=w384, name or relative path="TXT" ("名称或相对路径")) -> (appended path=w388:path)
            n230 = Build Path(base path=w388, name or relative path="SCD21-SDD21.txt" ("名称或相对路径")) -> (appended path=w386:path)
            n231 = local read "midVar_Content"() -> (w381:string)
            n232 = local read "Limit_SCD21-SDD21"() -> (w377:dbl[])
            n233 = call "xmlFull.vi"("single spec"=w377, "file path (dialog if empty)"=w386, "limit type"=enum16{"上限", "下限"}."上限", "SN"=w383, "数组"=string[] ["Port1-Port2: TD-RD", "Port1-Port2: RD-TD"], "second result"=w379) -> ("OutPutXml"=w385:string)  [unwired: 4 in]
            n234 = Concatenate Strings(w381, w385) -> (w380:string)
            n235 = local write "midVar_Content"(w380) -> ()
          }
          frame "body_e_SCD21-SDD21" {
            n236 = local read "midVar_Content"() -> (w394:string)
            n237 = Concatenate Strings(w394, "        </ItemTest>\n") -> (w393:string)
            n238 = local write "midVar_Content"(w393) -> ()
          }
          frame "body_s_paddle card" {
            n239 = local read "midVar_time"() -> (w402:string[])
            n240 = Index Array(array=w402, index #1=2 ("索引"), index #2=3 ("索引")) -> (element #1=w410:string, element #2=w407:string)
            n241 = local read "input_str_label"() -> (w401:string)
            n242 = Search and Replace String(input string="        <ItemTest ID=\"7\" name=\"Differential Impedance Paddle card\" startDateTime=\"@T1@\" endDateTime=\"@T2@\">\n            <TestResult BoardFlag=\"1\" ID=\"1\" SerialNumber=\"@L@\" ValueFlag=\"0\">\n                <Outcome value=\"@R@\"/>\n                <Description>NoDesc</Description>\n            </TestResult>\n ", search string="@T1@" ("搜索字符串"), replace string=w410) -> (result string=w409:string)  [unwired: 5 in, 3 out]
            n243 = Search and Replace String(input string=w409, search string="@T2@" ("搜索字符串"), replace string=w407) -> (result string=w405:string)  [unwired: 5 in, 3 out]
            n244 = Search and Replace String(input string=w405, search string="@L@" ("搜索字符串"), replace string=w401) -> (result string=w398:string)  [unwired: 5 in, 3 out]
            n245 = local read "TDD"() -> (w395:string)
            n246 = local read "midVar_Content"() -> (w400:string)
            n247 = Search and Replace String(input string=w398, search string="@R@" ("搜索字符串"), replace string=w395) -> (result string=w397:string)  [unwired: 5 in, 3 out]
            n248 = Concatenate Strings(w400, w397) -> (w399:string)
            n249 = local write "midVar_Content"(w399) -> ()
          }
          frame "body_detail_paddle card" {
            n250 = local read "txtPath"() -> (w439:path)
            n251 = Build Path(base path=w439, name or relative path="TXT" ("名称或相对路径")) -> (appended path=w442:path)
            n252 = local read "input_str_label"() -> (w436:string)
            n253 = local read "TDD"() -> (w417:string)
            n254 = Build Path(base path=w439, name or relative path="TXT" ("名称或相对路径")) -> (appended path=w447:path)
            n255 = local read "show_impspec"() -> (w416:string[])
            n256 = Build Path(base path=w442, name or relative path="TDD22.txt" ("名称或相对路径")) -> (appended path=w440:path)
            n257 = Build Path(base path=w447, name or relative path="TDD11.txt" ("名称或相对路径")) -> (appended path=w445:path)
            n258 = Index Array(array=w416, index=0 ("索引")) -> (element=w414:string)
            n259 = local read "midVar_Content"() -> (w420:string)
            n260 = local read "terminal points"() -> (w433:dbl[])
            n261 = Index Array(array=w433, index #1=0 ("索引"), index #2=1 ("索引")) -> (element #1=w424:dbl, element #2=w430:dbl)
            n262 = Subtract(x=w430, y=w424) -> (x-y=w427:dbl)
            n263 = Multiply(x=w427, y=0.1) -> (x*y=w426:dbl)
            n264 = Multiply(x=w427, y=0.2) -> (x*y=w425:dbl)
            n265 = Add(x=w424, y=w426) -> (x+y=w423:dbl)
            n266 = Add(x=w424, y=w425) -> (x+y=w422:dbl)
            n267 = Build Array(w423, w422) -> (w421:dbl[])
            n268 = call "xmlFull.vi"("TDD?"=TRUE, "Points"=w421, "file path (dialog if empty)"=w440, "TDD spec"=w414, "SN"=w436, "数组"=string[] ["Paddle Card_TD:ZDD22", "Paddle Card_RD:ZDD22"], "second result"=w417) -> ("OutPutXml"=w418:string)  [unwired: 3 in]
            n269 = call "xmlFull.vi"("TDD?"=TRUE, "Points"=w421, "file path (dialog if empty)"=w445, "TDD spec"=w414, "SN"=w436, "数组"=string[] ["Paddle Card_TD:ZDD11", "Paddle Card_RD:ZDD11"], "second result"=w417) -> ("OutPutXml"=w444:string)  [unwired: 3 in]
            n270 = Concatenate Strings(w420, w444, w418) -> (w419:string)
            n271 = local write "midVar_Content"(w419) -> ()
          }
          frame "body_e_paddle card" {
            n272 = local read "midVar_Content"() -> (w452:string)
            n273 = Concatenate Strings(w452, "        </ItemTest>\n") -> (w451:string)
            n274 = local write "midVar_Content"(w451) -> ()
          }
          frame "body_s_ILD" {
            n275 = local read "midVar_time"() -> (w459:string[])
            n276 = Index Array(array=w459, index #1=3 ("索引"), index #2=4 ("索引")) -> (element #1=w470:string, element #2=w467:string)
            n277 = Search and Replace String(input string="        <ItemTest ID=\"8\" name=\"Insertion Loss Deviation\" startDateTime=\"@T1@\" endDateTime=\"@T2@\">\n            <TestResult BoardFlag=\"1\" ID=\"1\" SerialNumber=\"@L@\" ValueFlag=\"0\">\n                <Outcome value=\"@R@\"/>\n                <Description>NoDesc</Description>\n            </TestResult>\n ", search string="@T1@" ("搜索字符串"), replace string=w470) -> (result string=w469:string)  [unwired: 5 in, 3 out]
            n278 = Search and Replace String(input string=w469, search string="@T2@" ("搜索字符串"), replace string=w467) -> (result string=w462:string)  [unwired: 5 in, 3 out]
            n279 = local read "input_str_label"() -> (w461:string)
            n280 = local read "ILD"() -> (w454:string)
            n281 = Search and Replace String(input string=w462, search string="@L@" ("搜索字符串"), replace string=w461) -> (result string=w457:string)  [unwired: 5 in, 3 out]
            n282 = local read "midVar_Content"() -> (w466:string)
            n283 = Search and Replace String(input string=w457, search string="@R@" ("搜索字符串"), replace string=w454) -> (result string=w456:string)  [unwired: 5 in, 3 out]
            n284 = Concatenate Strings(w466, w456) -> (w465:string)
            n285 = local write "midVar_Content"(w465) -> ()
          }
          frame "body_detail_ILD" {
            n286 = local read "txtPath"() -> (w481:path)
            n287 = Build Path(base path=w481, name or relative path="TXT" ("名称或相对路径")) -> (appended path=w485:path)
            n288 = local read "input_str_label"() -> (w479:string)
            n289 = local read "ILD"() -> (w476:string)
            n290 = local read "Limit_ILD"() -> (w473:dbl[])
            n291 = local read "midVar_Content"() -> (w477:string)
            n292 = Build Path(base path=w485, name or relative path="ILD.txt" ("名称或相对路径")) -> (appended path=w483:path)
            n293 = call "xmlFull.vi"("single spec"=w473, "file path (dialog if empty)"=w483, "limit type"=enum16{"上限", "下限"}."上限", "SN"=w479, "ABS?"=TRUE, "数组"=string[] ["Port1-Port2: TD-RD", "Port1-Port2: RD-TD"], "second result"=w476) -> ("OutPutXml"=w482:string)  [unwired: 3 in]
            n294 = Concatenate Strings(w477, w482) -> (w478:string)
            n295 = local write "midVar_Content"(w478) -> ()
          }
          frame "body_e_ILD" {
            n296 = local read "midVar_Content"() -> (w491:string)
            n297 = Concatenate Strings(w491, "        </ItemTest>\n") -> (w490:string)
            n298 = local write "midVar_Content"(w490) -> ()
          }
          frame "tail" {
            # "</ResultSet>\n    <TestProgram Productline=\"XT-113\" Product=\"SFP+\">\n        <c:Definition name=\"HPTS\" version=\"6.0\">\n            <c:Description>NoDesc</c:Description> \n        </c:Definition>\n    </TestProgram>\n    <!--  ATE--> \n    <TestStation AteName=\"TDR\" AteVersion=\"1.001\" /> \n    <!--  SerialNumber--> \n    <UUT UutType=\"hardware\">\n        <SerialNumber>@L@</SerialNumber> \n        <ItemName>SFP+</ItemName>\n        <ItemCode>@C@</ItemCode> \n    </UUT>\n    <WorkOrder>\n        <WorkItem name=\"a\">\n            <c:Datum xsi:type=\"c:string\">\n                <c:Value>SPZS06311C1</c:Value> \n            </c:Datum>\n        </WorkItem>\n    </WorkOrder>\n</TestResults"
            n299 = local read "FileVer"() -> (w493:string)
            n300 = Concatenate Strings("\"" ("字符串"), w493, "\"" ("字符串")) -> (w498:string)
            n301 = local read "FilePath"() -> (w492:string)
            n302 = local read "input_str_product"() -> (w518:string)
            n303 = Search and Replace String(input string="    </ResultSet>\n    <TestProgram Productline=\"XT-113\" Product=\"SFP+\">\n        <c:Definition name=\"VNA\" version=@Ver@>\n            <c:Description>@Path@</c:Description> \n        </c:Definition>\n    </TestProgram>\n    <!--  ATE--> \n    <TestStation AteName=@PCName@ AteVersion=\"1.001\" /> \n    <!--  SerialNumber--> \n    <UUT UutType=\"hardware\">\n        <SerialNumber>@L@</SerialNumber> \n        <ItemName>SFP+</ItemName>\n        <ItemCode>@C@</ItemCode> \n    </UUT>\n    <WorkOrder>\n        <WorkItem name=\"a\">\n            <c:Datum xsi:type=\"c:string\">\n                <c:Value>SPZS06311C1</c:Value> \n            </c:Datum>\n        </WorkItem>\n    </WorkOrder>\n</TestResults>", search string="@Ver@" ("搜索字符串"), replace string=w498) -> (result string=w505:string)  [unwired: 5 in, 3 out]
            n304 = call "PCsName.vi"() -> ("Computer Name"=w497:string)
            n305 = Search and Replace String(input string=w505, search string="@Path@" ("搜索字符串"), replace string=w492) -> (result string=w503:string)  [unwired: 5 in, 3 out]
            n306 = local read "input_str_label"() -> (w515:string)
            n307 = Concatenate Strings("\"" ("字符串"), w497, "\"" ("字符串")) -> (w494:string)
            n308 = Search and Replace String(input string=w503, search string="@PCName@" ("搜索字符串"), replace string=w494) -> (result string=w501:string)  [unwired: 5 in, 3 out]
            n309 = Search and Replace String(input string=w501, search string="@P@" ("搜索字符串"), replace string=w518) -> (result string=w517:string)  [unwired: 5 in, 3 out]
            n310 = Search and Replace String(input string=w517, search string="@L@" ("搜索字符串"), replace string=w515) -> (result string=w510:string)  [unwired: 5 in, 3 out]
            n311 = local read "input_str_CustomerPN"() -> (w508:string)
            n312 = local read "midVar_Content"() -> (w514:string)
            n313 = Search and Replace String(input string=w510, search string="@C@" ("搜索字符串"), replace string=w508) -> (result string=w511:string)  [unwired: 5 in, 3 out]
            n314 = Concatenate Strings(w514, w511) -> (w513:string)
            n315 = local write "midVar_Content"(w513) -> ()
          }
          frame "end" {
            n316 = local read "midVar_Content"() -> (w521:string)
            n317 = Open/Create/Replace File(file path (use dialog)="xmlPath", operation (0:open)=T4."open or create" ("操作(0:open)")) -> (refnum out=w525:refnum<file>)  [unwired: 4 in, 2 out]
            n318 = Text to UTF-8(11:w521) -> (3:w520:string)  [unwired: 1 in, 1 out]
            n319 = Write to Text File(file (use dialog)=w525, text=w520) -> (refnum out=w524:refnum<file>)  [unwired: 2 in, 2 out]
            n320 = Close File(refnum=w524) -> ()  [unwired: 1 in, 2 out]
          }
        }
        n321 = local write "midVar_state"(w70) -> ()
      }
    }
  }
